vi "PH_Revolver-GUI_6P.destructor.vi"(0 "i ref in":refnum<vi>, 5 "error in(no error)":errorcluster) -> (19 "error out":errorcluster)   [LabVIEW 2014, in "PH_Revolver-GUI_6P.lvlib"]
doc: "This is the destructor of a class.\n\nLicense Agreement for this software:\n\nCopyright (C)\nGesellschaft für Schwerionenforschung, GSI\nPlanckstr. 1\n64291 Darmstadt\nGermany\n\nContact: D.Beck@gsi.de \n\nThis program is free software; you can redistribute it and/or modify it under the terms of the \nGNU General Public License as published by the Free Software Foundation; either version 2 of \nthe license, or (at your option) any later version.\n\nThis program is distributed in the hope that it will be useful, but WITHOUT ANY WARRANTY; \nwithout even the implied warranty of MERCHANTABILITY or FITNESS FOR A PARTICULAR PURPOSE. See the GNU General License for more details (http://www.gnu.org).\n\nGesellschaft für Schwerionenforschung, GSI\nPlanckstr. 1, 64291 Darmstadt, Germany\nFor all questions and ideas contact: M.Richter@gsi.de, H.Brand@gsi.de or D.Beck@gsi.de.\nLast update: 16-JUN-2004"
uses:
  PH_Revolver-GUI_6P.lvlib
  lib.lib/DimLVEvent/LVDimInterface/LVDimInterface.lvlib
  PH_PSDBWriter/PH_PSDBWriter.lvlib
  PH_AxisGUI_BaseClass/PH_AxisGUI_BaseClass.lvlib
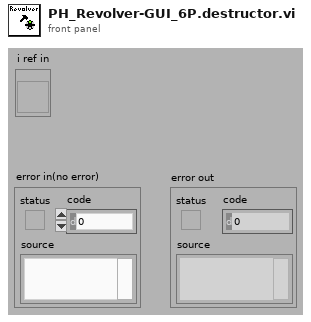
[diagram p1: front panel]
types:
  T1 = typedef "PH_Revolver-GUI_6P.lvlib/PH_Revolver-GUI_6P.i attribute.ctl" = cluster{"GUI Refs":cluster{"0°":refnum<vi>, "60°":refnum<vi>, "120°":refnum<vi>, "180°":refnum<vi>, "240°":refnum<vi>, "300°":refnum<vi>, "Action":refnum<vi>}, "Revolver Position":T2, "Service ID Position":i32, "Captions":string[]}
  T2 = typedef "PH_Revolver-GUI_6P.lvlib/PH_Revolver-GUI_6P.Position.ctl" = u16
  T3 = enum16{"SetAttribute", "GetAttribute", "CreateAttribute", "DestroyAttribute", "DestroyAllAtributes"}
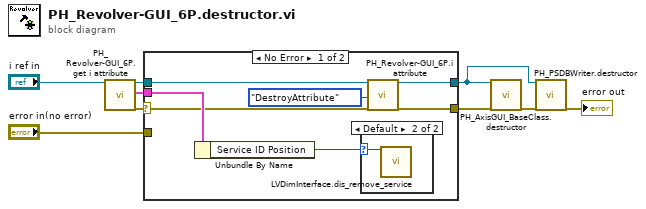
[diagram p0: block diagram]
diagram:
  n1 = call "PH_Revolver-GUI_6P.get i attribute.vi"("i ref in"="i ref in") -> ("i ref out"=w7:refnum<vi>, "i attribute"=w8:T1, "error out"=w5:errorcluster)  [unwired: 16 in]
  n2 = case shown="No Error" w5 {
    selector: w5 -> [w10 _]
    tunnel: w8 -> [w14 _]
    tunnel: [w13 w18] -> w3
    tunnel: w7 -> [w12 w19]
    tunnel: [w11 w19] -> w6
    tunnel: "error in(no error)" -> [_ w18]
    frame No Error {
      n3 = Unbundle By Name(w14) -> ("Service ID Position"=w15:i32)
      n4 = case shown="Default" w15 {
        selector: w15 -> [_ w17]
        frame -1 {
        }
        frame Default {
          n5 = call "LVDimInterface.dis_remove_service.vi"("my_serviceID"=w17) -> ()  [unwired: 18 in, 1 out]
        }
      }
      n6 = call "PH_Revolver-GUI_6P.i attribute.vi"("VI Refnum"=w12, "Action"=T3."DestroyAttribute", "error in (no error)"=w10) -> ("VI Refnum out"=w11:refnum<vi>, "error out"=w13:errorcluster)  [unwired: 14 in, 1 out]
    }
    frame Error {
    }
  }
  n7 = call "PH_AxisGUI_BaseClass.destructor.vi"("i ref in"=w6, "error in(no error)"=w3) -> ("error out"=w2:errorcluster)  [unwired: 17 in]
  n8 = call "PH_PSDBWriter.destructor.vi"("i ref in"=w6, "error in(no error)"=w2) -> ("error out"=→"error out":errorcluster)  [unwired: 17 in]
